vi "PH_AxisGUI_BaseClass.PC_Information.vi"(0 "i ref in":refnum<vi>, 2 "Service Name":string="N/A", 3 "Axis Information":T1, 4 "no link":bool, 5 "error in":errorcluster) -> (14 "i ref out":refnum<vi>, 16 "Axis":i32=-1, 19 "error out":errorcluster)   [LabVIEW 2014, in "PH_AxisGUI_BaseClass.lvlib"]
doc: "This VI deals with information given by an axis."
uses:
  PH_AxisGUI_BaseClass.lvlib
  PH_Stepmotor_BaseClass/PH_Stepmotor_BaseClass.Axis Information.ctl
  PH_Stepmotor_BaseClass/PH_Stepmotor_BaseClass.Axis Activity.ctl
  PH_Stepmotor_BaseClass/PH_Stepmotor_BaseClass.Axis DIM Tags.ctl
  PH_StatusHandler/PH_StatusHandler.Status.ctl
  PH_Stepmotor_BaseClass/PH_Stepmotor_BaseClass.lvlib
  PH_StatusHandler/PH_StatusHandler.lvlib
  PH_Common/PH_Common.lvlib
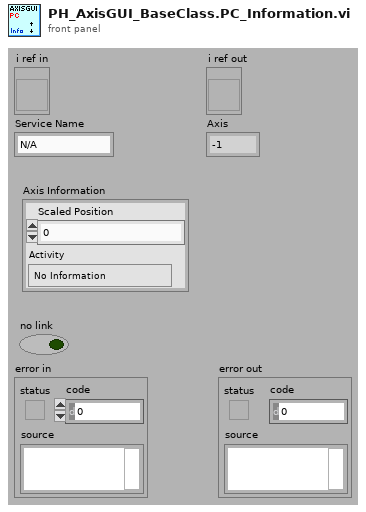
[diagram p1: front panel]
types:
  T1 = typedef "PH_Stepmotor_BaseClass.lvlib/PH_Stepmotor_BaseClass.Axis Information.ctl" = cluster{"Scaled Position":dbl, "Activity":T2}
  T2 = typedef "PH_Stepmotor_BaseClass.lvlib/PH_Stepmotor_BaseClass.Axis Activity.ctl" = enum16{"No Information", "stopped", "running", "Failure", "Alarm", "stopped at backward ES", "stopped at foreward ES"}
  T3 = typedef "PH_Stepmotor_BaseClass.lvlib/PH_Stepmotor_BaseClass.Axis DIM Tags.ctl" = enum16{"no Info", "Information", "Settings"}
  T4 = enum8{"Enabled", "Disabled", "Disabled and Grayed Out"}
  T5 = typedef "PH_AxisGUI_BaseClass.lvlib/PH_AxisGUI_BaseClass.i attribute.ctl" = cluster{"Axes":T6[]}
  T6 = typedef "PH_AxisGUI_BaseClass.lvlib/PH_AxisGUI_BaseClass.Axis Attributes.ctl" = cluster{"Axis GUI Refs":T7, "Address":T8, "Name":string, "Label \"Back\"":string, "Labell \"Forth\"":string, "Moving?":bool}
  T7 = typedef "PH_AxisGUI_BaseClass.lvlib/PH_AxisGUI_BaseClass.Axis GUI Refs.ctl" = cluster{"Back":refnum<vi>, "Forth":refnum<vi>, "Status":refnum<vi>, "Target":refnum<vi>, "Address":refnum<vi>, "Status Bar":refnum<vi>, "Settings":refnum<vi>, "Activity":refnum<vi>, "Clear Error":refnum<vi>}
  T8 = typedef "PH_Stepmotor_BaseClass.lvlib/PH_Stepmotor_BaseClass.Axis Address.ctl" = cluster{"Instance":string, "Motor Nr":i32}
  T9 = typedef "PH_StatusHandler.lvlib/PH_StatusHandler.Status.ctl" = i16
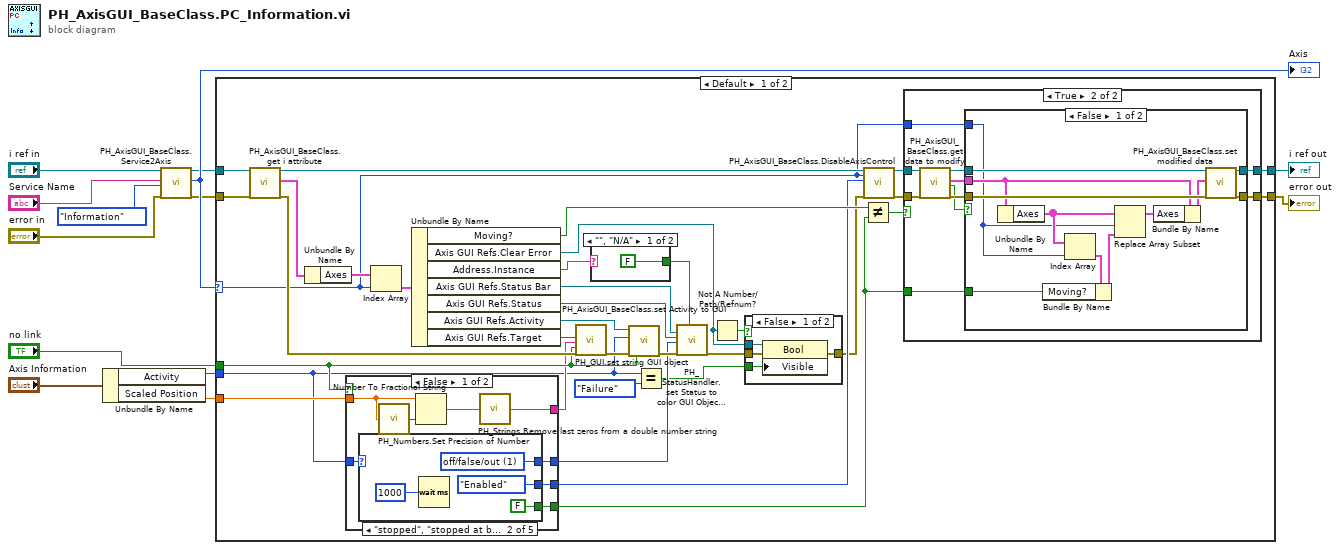
[diagram p0: block diagram]
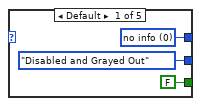
[diagram p3: hidden frame]
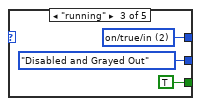
[diagram p4: hidden frame]
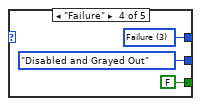
[diagram p5: hidden frame]
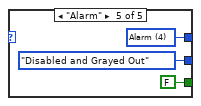
[diagram p6: hidden frame]
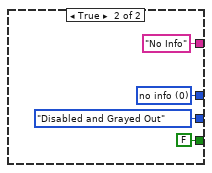
[diagram p7: hidden frame]
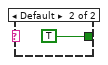
[diagram p10: hidden frame]
diagram:
  n1 = Unbundle By Name("Axis Information") -> ("Activity"=w3:T2, "Scaled Position"=w1:dbl)
  n2 = call "PH_AxisGUI_BaseClass.Service2Axis.vi"("i ref in"="i ref in", "Service Name"="Service Name", "Tag"=PH_Stepmotor_BaseClass.Axis_DIM_Tags."Information", "error in"="error in") -> ("i ref out"=w8:refnum<vi>, "Axis"=w9:i32, "error out"=w7:errorcluster)  [unwired: 12 in, 1 out]
  "Axis" <- w9
  n3 = case shown="Default" w9 {
    selector: w9 -> [w23 _]
    tunnel: w8 -> [w35 w111]
    tunnel: w7 -> [w34 w110]
    tunnel: [w32 w111] -> w5
    tunnel: [w33 w110] -> w6
    tunnel: w1 -> [w25 _]
    tunnel: w3 -> [w18 _]
    tunnel: "no link" -> [w29 _]
    frame Default {
      n4 = call "PH_AxisGUI_BaseClass.get i attribute.vi"("i ref in"=w35, "error in (no error)"=w34) -> ("i ref out"=w46:refnum<vi>, "i attribute"=w48:T5, "error out"=w36:errorcluster)  [unwired: 15 in]
      n5 = Unbundle By Name(w48) -> ("Axes"=w47:T6[])
      n6 = case shown="False" w29 {
        tunnel: w18 -> [w61 _]
        tunnel: [w60 w81] -> w28
        tunnel: [w59 T4."Disabled and Grayed Out" ("f")] -> w27
        tunnel: [w56 "No Info"] -> w26
        tunnel: w25 -> [w55 _]
        tunnel: [w57 FALSE] -> w24
        frame False {
          n7 = case shown="\"stopped\", \"stopped at backward ES\", \"stopped at foreward ES\"" w61 {
            tunnel: [w64 w68 w71 w74 w77] -> w60
            tunnel: [T4."Disabled and Grayed Out" ("f") T4."Enabled" ("f") T4."Disabled and Grayed Out" ("f") T4."Disabled and Grayed Out" ("f") T4."Disabled and Grayed Out" ("f")] -> w59
            tunnel: [FALSE FALSE TRUE FALSE FALSE] -> w57
            frame Default {
              w64 = T9 0 items=["no info", "off/false/out", "on/true/in", "Failure", "Alarm", "Status 1", "Status 2", "Status 3"] ("State")
            }
            frame "stopped", "stopped at backward ES", "stopped at foreward ES" {
              w68 = T9 1 items=["no info", "off/false/out", "on/true/in", "Failure", "Alarm", "Status 1", "Status 2", "Status 3"] ("State")
              n8 = Wait (ms)(milliseconds to wait=u32 1000) -> ()  [unwired: 1 out]
            }
            frame "running" {
              w71 = T9 2 items=["no info", "off/false/out", "on/true/in", "Failure", "Alarm", "Status 1", "Status 2", "Status 3"] ("State")
            }
            frame "Failure" {
              w74 = T9 3 items=["no info", "off/false/out", "on/true/in", "Failure", "Alarm", "Status 1", "Status 2", "Status 3"] ("State")
            }
            frame "Alarm" {
              w77 = T9 4 items=["no info", "off/false/out", "on/true/in", "Failure", "Alarm", "Status 1", "Status 2", "Status 3"] ("State")
            }
          }
          n9 = call "PH_Numbers.Set Precision of Number.vi"("Number"=w55) -> ("Precision"=w54:i16)
          n10 = Number To Fractional String(number=w55, precision (6)=w54) -> (F-format string=w58:string)  [unwired: 2 in]
          n11 = call "PH_Strings.Remove last zeros from a double number string.vi"("String in"=w58) -> ("String out"=w56:string)
        }
        frame True {
          w81 = T9 0 items=["no info", "off/false/out", "on/true/in", "Failure", "Alarm", "Status 1", "Status 2", "Status 3"] ("State")
        }
      }
      n12 = Index Array(array=w47, index=w23) -> (element=w45:T6)
      n13 = Unbundle By Name(w45) -> ("Moving?"=w31:bool, "Axis GUI Refs.Clear Error"=w14:refnum<vi>, "Address.Instance"=w15:string, "Axis GUI Refs.Status Bar"=w41:refnum<vi>, "Axis GUI Refs.Status"=w42:refnum<vi>, "Axis GUI Refs.Activity"=w38:refnum<vi>, "Axis GUI Refs.Target"=w37:refnum<vi>)
      n14 = call "PH_GUI.set string GUI object.vi"("GUI object Ref"=w37, "Text"=w26, "Blinking? (false)"=w29, "error in"=w36) -> ("error out"=w40:errorcluster)  [unwired: 15 in]
      n15 = case shown="\"\", \"N/A\"" w15 {
        tunnel: [FALSE TRUE] -> w44
        frame "", "N/A" {
        }
        frame Default {
        }
      }
      n16 = call "PH_AxisGUI_BaseClass.set Activity to GUI.vi"("error in"=w40, "no link"=w29, "Activity"=w18, "GUI Ref Activity"=w38) -> ("error out"=w39:errorcluster)  [unwired: 3 in]
      n17 = Equal?(x=w18, y=PH_Stepmotor_BaseClass.Axis_Activity."Failure") -> (x = y?=w16:bool)
      n18 = call "PH_StatusHandler.set Status to color GUI Object for Color Blinds.vi"("Ref CB State"=w41, "Ref State"=w42, "State"=w28, "error in"=w39, "Visible? (true)"=w44) -> ("error out"=w43:errorcluster)  [unwired: 14 in]
      n19 = Not A Number/Path/Refnum?(number/path/refnum=w14) -> (NaN/Path/Refnum?=w19:bool)
      n20 = case shown="False" w19 {
        tunnel: w43 -> [w52 w53]
        tunnel: [w51 w53] -> w20
        tunnel: w14 -> [w50 _]
        tunnel: w16 -> [w49 _]
        frame False {
          n21 = property class="Bool"(reference=w50, error in=w52, "Visible"=w49) -> (error out=w51:errorcluster)  [unwired: 1 out]
        }
        frame True {
        }
      }
      n22 = Not Equal?(x=w31, y=w24) -> (x != y?=w30:bool)
      n23 = call "PH_AxisGUI_BaseClass.DisableAxisControl.vi"("i ref in"=w46, "Axis"=w23, "Disabled"=w27, "error in"=w20) -> ("i ref out"=w22:refnum<vi>, "error out"=w21:errorcluster)  [unwired: 14 in]
      n24 = case shown="True" w30 {
        tunnel: w21 -> [w82 w93]
        tunnel: [w82 w91] -> w33
        tunnel: w22 -> [w83 w90]
        tunnel: [w83 w88] -> w32
        tunnel: w23 -> [_ w85]
        tunnel: w24 -> [_ w84]
        frame False {
        }
        frame True {
          n25 = call "PH_AxisGUI_BaseClass.get data to modify.vi"("i ref in"=w90, "error in (no error)"=w93) -> ("i ref out"=w89:refnum<vi>, "i attribute"=w86:T5, "timed out"=w87:bool, "error out"=w92:errorcluster)  [unwired: 14 in]
          n26 = case shown="False" w87 {
            tunnel: w92 -> [w105 w106]
            tunnel: [w104 w106] -> w91
            tunnel: w89 -> [w103 w107]
            tunnel: [w102 w107] -> w88
            tunnel: w86 -> [w100 _]
            tunnel: w85 -> [w96 _]
            tunnel: w84 -> [w94 _]
            frame False {
              n27 = Unbundle By Name(w100) -> ("Axes"=w98:T6[])
              n28 = Index Array(array=w98, index=w96) -> (element=w97:T6)
              n29 = Bundle By Name(cluster=w97, "Moving?"=w94) -> (w95:T6)
              n30 = Replace Array Subset(array=w98, new element=w95, index=w96) -> (w99:T6[])
              n31 = Bundle By Name(cluster=w100, "Axes"=w99) -> (w101:T5)
              n32 = call "PH_AxisGUI_BaseClass.set modified data.vi"("i ref in"=w103, "i attribute"=w101, "error in (no error)"=w105) -> ("i ref out"=w102:refnum<vi>, "error out"=w104:errorcluster)  [unwired: 15 in]
            }
            frame True {
            }
          }
        }
      }
    }
    frame -1 {
    }
  }
  "error out" <- w6
  "i ref out" <- w5
